vi "itc 503 box controller -- A0.vi"(6 "Log File Path":path, 7 "itc box action":T2=enum."read sweep table", 8 "error in":errorcluster, 9 "Sweep Table In":dbl[][](array[numeric])=[[650.0, 1334.0, 30.0], [300.0, 1334.0, 0.0], [0.0, 0.0, 0.0], [0.0, 0.0, 0.0], [0.0, 0.0, 0.0], [0.0, 0.0, 0.0], [0.0, 0.0, 0.0], [0.0, 0.0, 0.0], [0.0, 0.0, 0.0], [0.0, 0.0, 0.0], [0.0, 0.0, 0.0], [300.0, 0.0, 0.0], [0.0, 0.0, 0.0], [0.0, 0.0, 0.0], [0.0, 0.0, 0.0], [300.0, 0.0, 0.0]], 10 "input":dbl=300.0, 11 "VISA resource name":refnum<visa-resource-name>="GPIB0::23::INSTR") -> (0 "error out":errorcluster, 1 "Sweep Table":dbl[][](array[numeric])=[[650.0, 1334.0, 30.0], [300.0, 1334.0, 0.0], [0.0, 0.0, 0.0], [0.0, 0.0, 0.0], [0.0, 0.0, 0.0], [0.0, 0.0, 0.0], [0.0, 0.0, 0.0], [0.0, 0.0, 0.0], [0.0, 0.0, 0.0], [0.0, 0.0, 0.0], [0.0, 0.0, 0.0], [300.0, 0.0, 0.0], [0.0, 0.0, 0.0], [0.0, 0.0, 0.0], [0.0, 0.0, 0.0], [300.0, 0.0, 0.0]], 2 "itc box state OUT":T1={"ITC503 Address"="GPIB0::15::INSTR", "ITC temperature"=0.0, "ITC set temperature"=300.0, "heater"=300.0, "gas flow"=1.6, "P"=0.0, "D"=10.0, "I"=0.1, "ITC state"="X0A1C2S01H1L0\r", "nonzero temperature"=0.0, "Magn Field (T)"=0.0})   [LabVIEW 2015]
uses:
  itc 503 box - control.ctl
  itc 503 box state.ctl
  Q - not nan -- real.vi
panel:
  out "F-format string":string
  out "enabled state":enum16{"disabled", "enabled"}(ring)
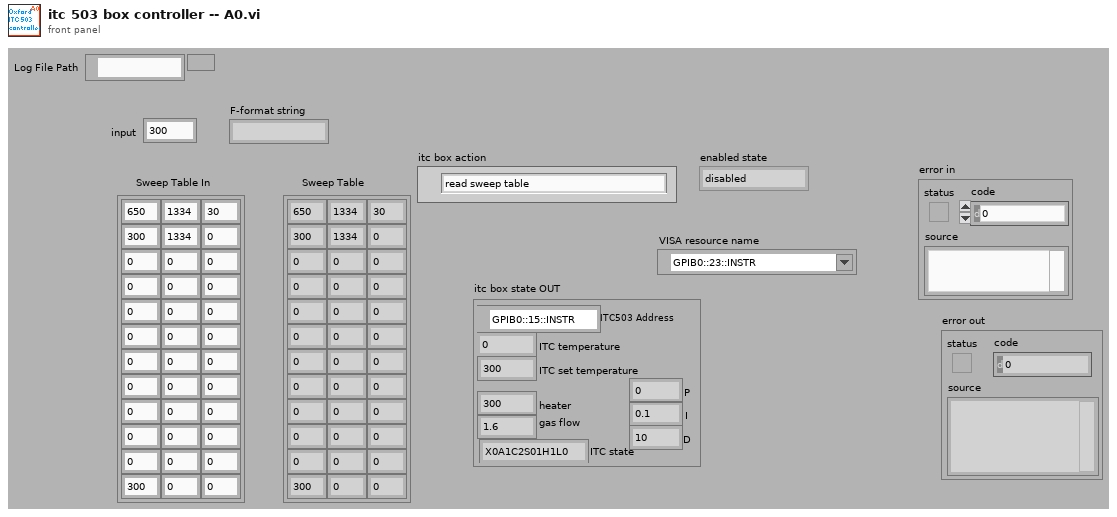
[diagram p1: front panel]
types:
  T1 = typedef "itc 503 box state.ctl" = cluster{"ITC503 Address":refnum<visa-resource-name>, "ITC temperature":dbl, "ITC set temperature":dbl, "heater":dbl, "gas flow":dbl, "P":dbl, "D":dbl, "I":dbl, "ITC state":string, "nonzero temperature":dbl, "Magn Field (T)":dbl}
  T2 = typedef "itc 503 box - control.ctl" = enum16{"heater manual and zero", "heater auto", "upload D", "upload I", "upload P", "shut off", "init", "read sweep table", "disable", "enable", "read state", "set gas to", "stop sweep", "start sweep", "test", "set temperature to", "write sweep table", "-void", "set heater to"}
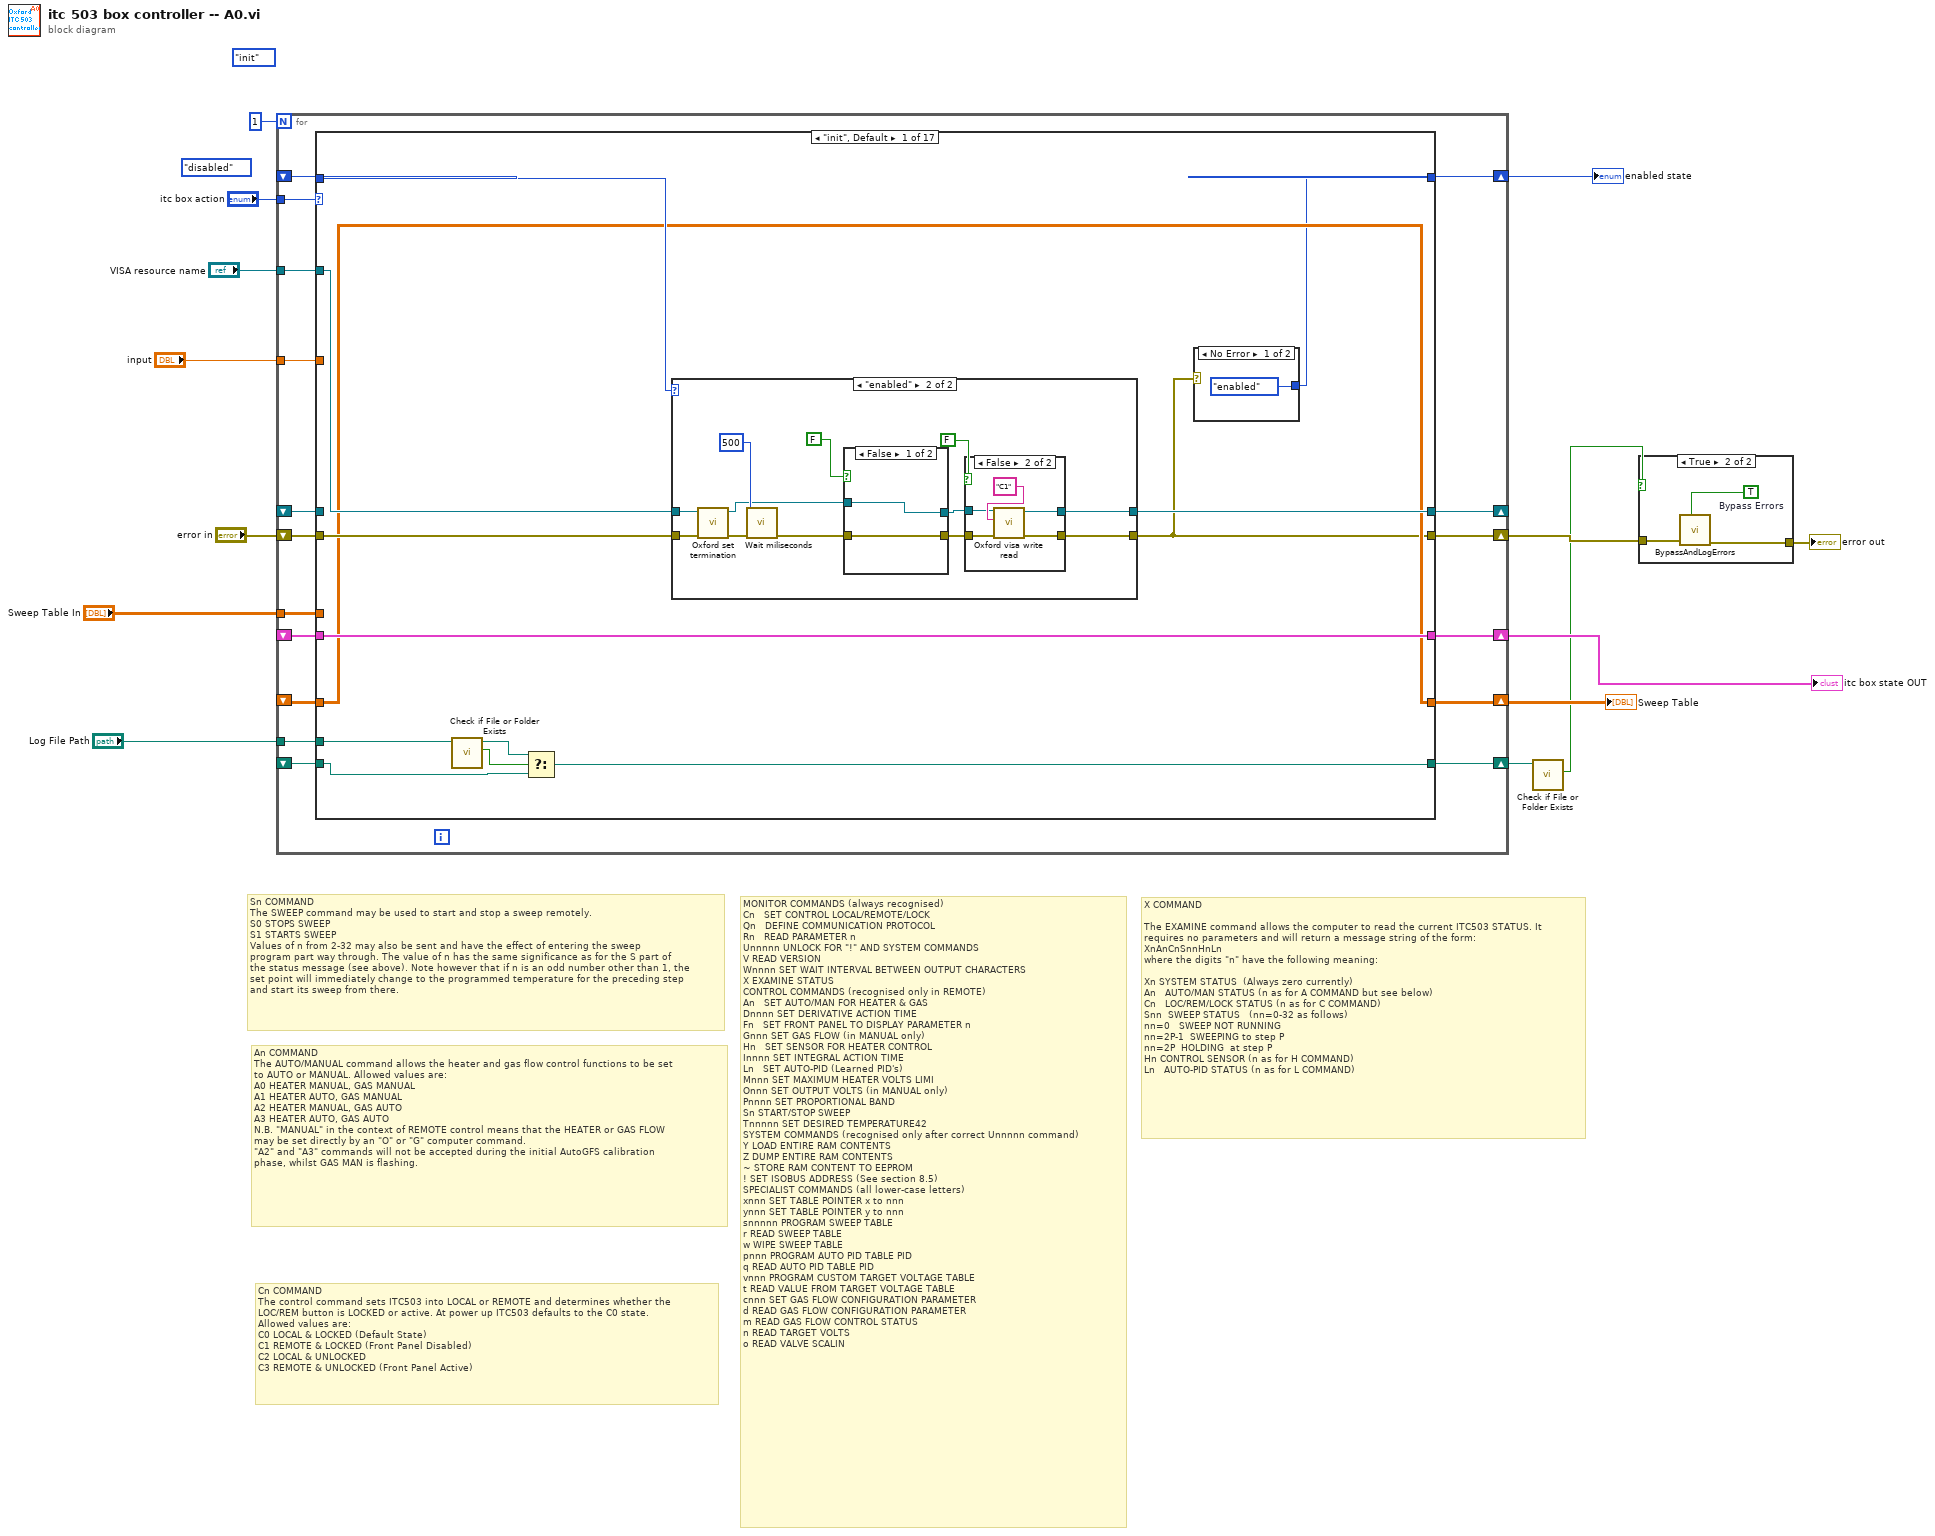
[diagram p0: block diagram]
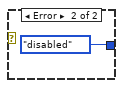
[diagram p3: hidden frame]
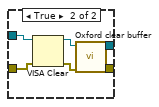
[diagram p5: hidden frame]
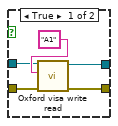
[diagram p6: hidden frame]
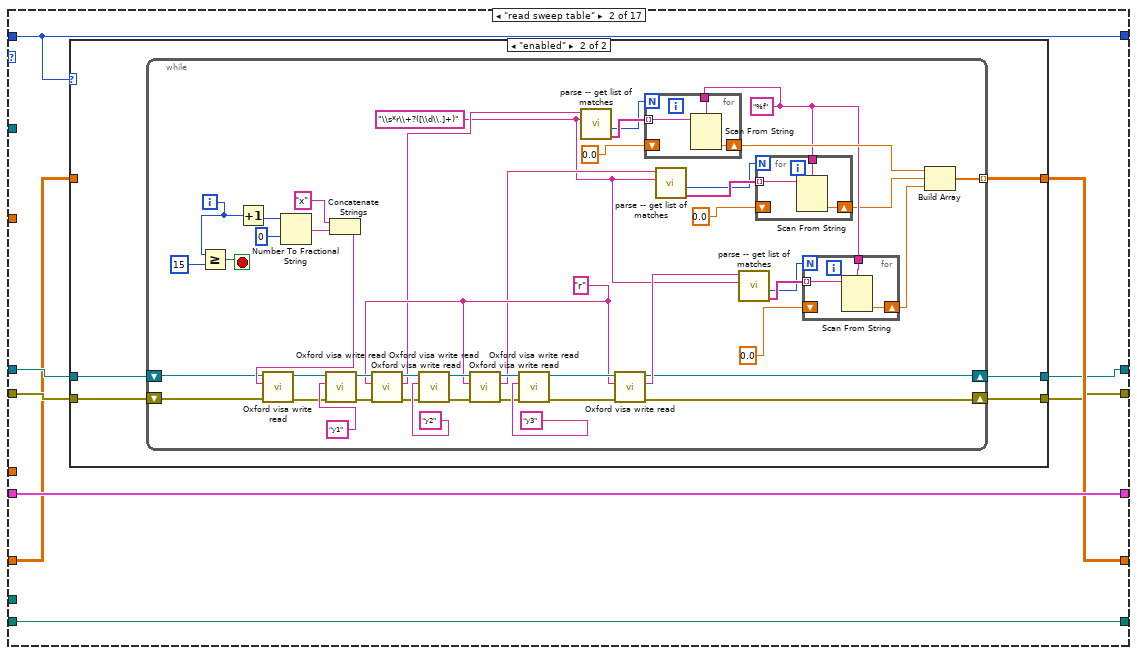
[diagram p7: hidden frame]
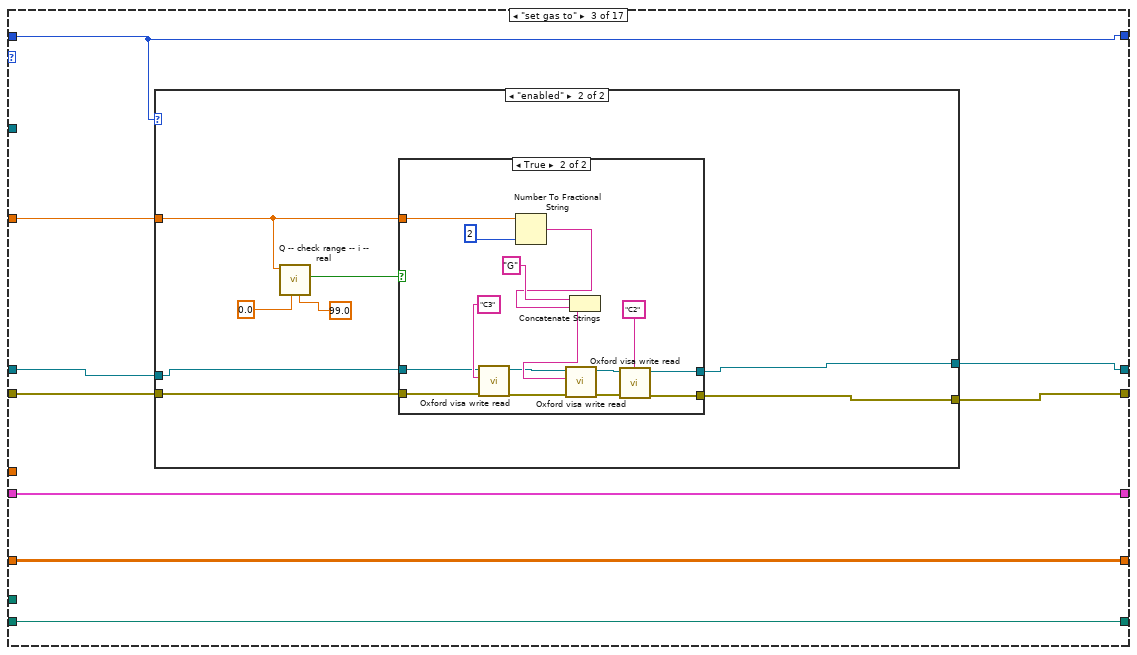
[diagram p9: hidden frame]
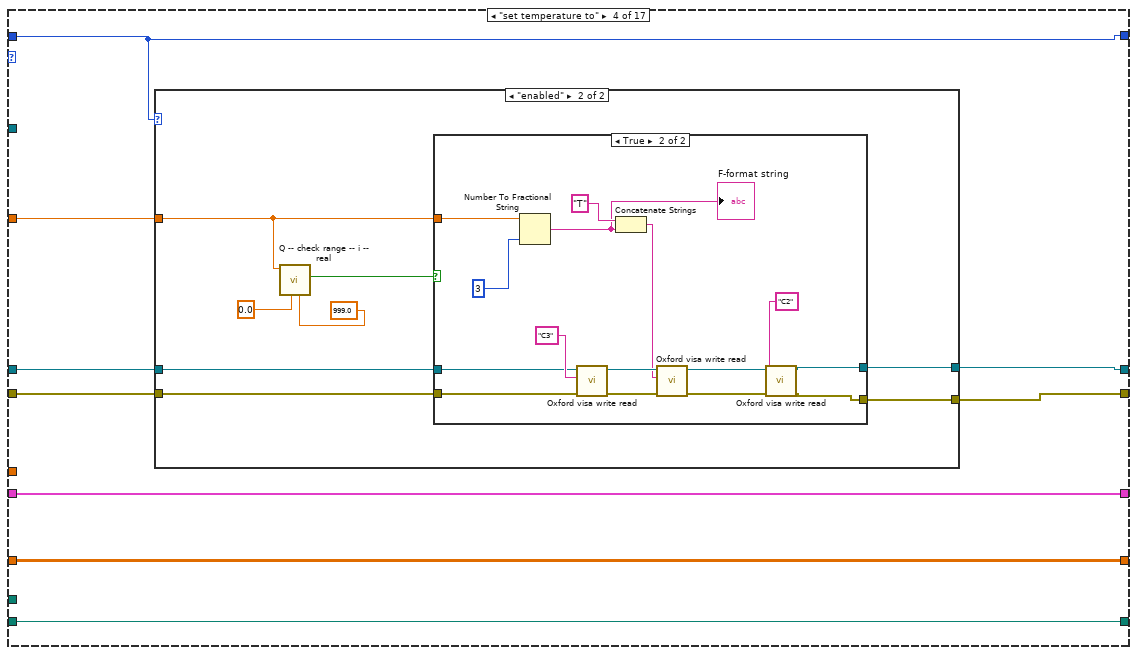
[diagram p12: hidden frame]
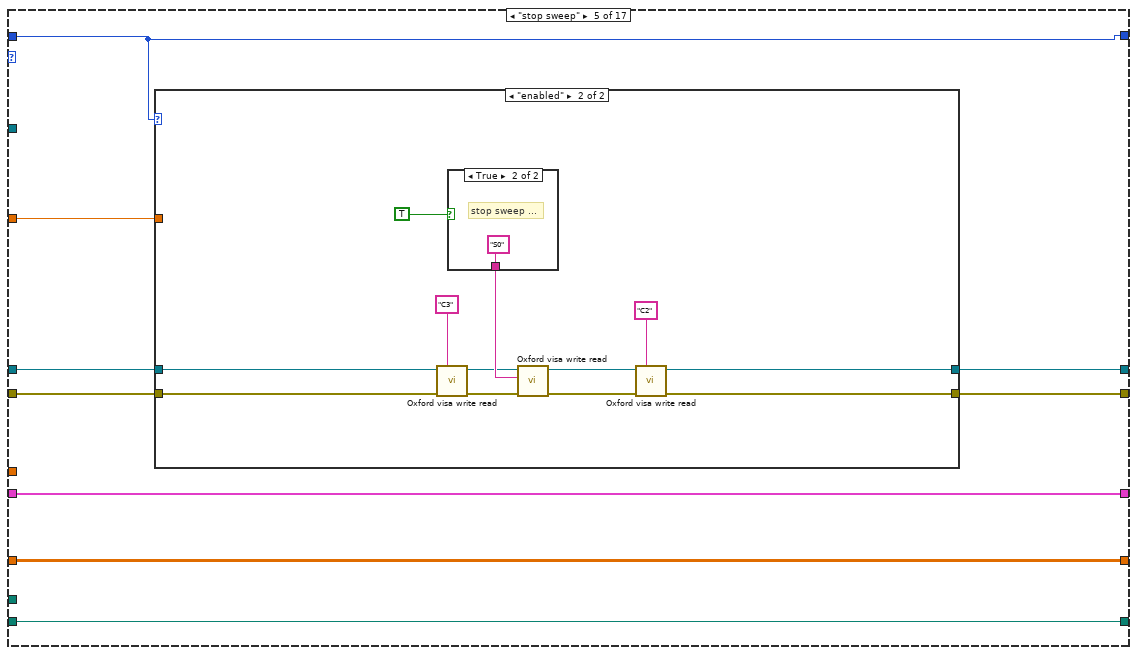
[diagram p15: hidden frame]
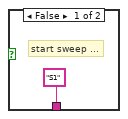
[diagram p17: hidden frame]
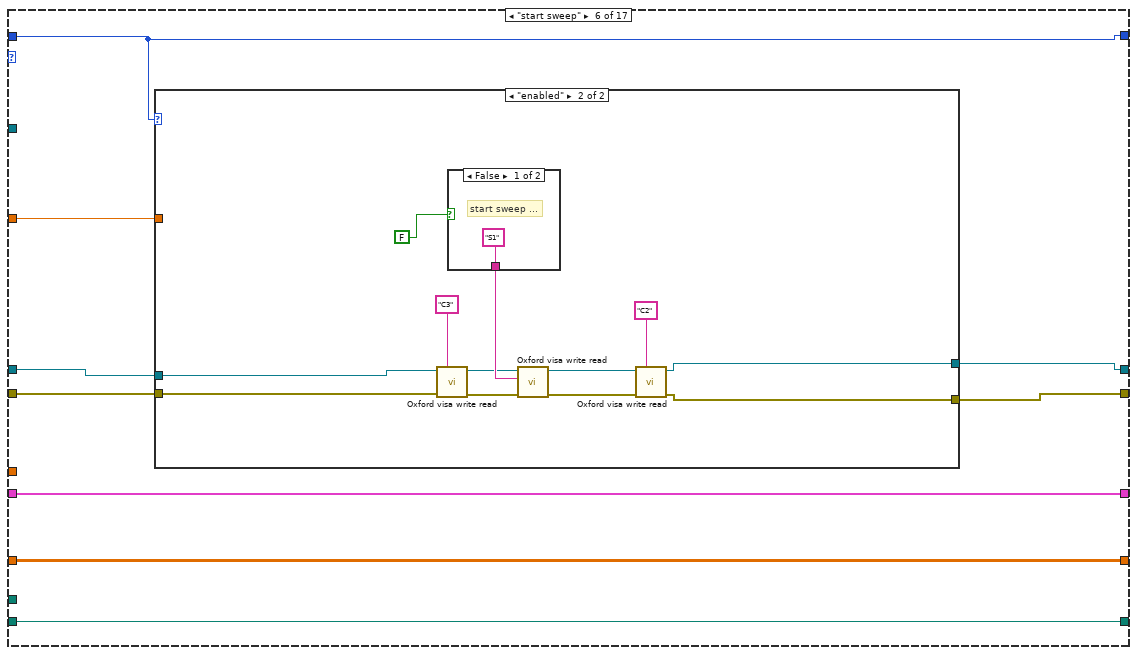
[diagram p18: hidden frame]
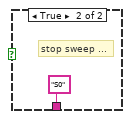
[diagram p20: hidden frame]
diagram:
  (unwired) enum16{"disabled", "enabled"}."disabled" ("disable interaction with itc  2")
  (unwired) itc_503_box_-_control."init" ("itc box action")
  # "Cn COMMAND\nThe control command sets ITC503 into LOCAL or REMOTE and determines whether the\nLOC/REM button is LOCKED or active. At power up ITC503 defaults to the C0 state.\nAllowed values are:\nC0 LOCAL & LOCKED (Default State)\nC1 REMOTE & LOCKED (Front Panel Disabled)\nC2 LOCAL & UNLOCKED\nC3 REMOTE & UNLOCKED (Front Panel Active)"
  # "An COMMAND\nThe AUTO/MANUAL command allows the heater and gas flow control functions to be set\nto AUTO or MANUAL. Allowed values are:\nA0 HEATER MANUAL, GAS MANUAL\nA1 HEATER AUTO, GAS MANUAL\nA2 HEATER MANUAL, GAS AUTO\nA3 HEATER AUTO, GAS AUTO\nN.B. \"MANUAL\" in the context of REMOTE control means that the HEATER or GAS FLOW\nmay be set directly by an \"O\" or \"G\" computer command.\n\"A2\" and \"A3\" commands will not be accepted during the initial AutoGFS calibration\nphase, whilst GAS MAN is flashing."
  # "MONITOR COMMANDS (always recognised)\nCn   SET CONTROL LOCAL/REMOTE/LOCK\nQn   DEFINE COMMUNICATION PROTOCOL\nRn   READ PARAMETER n\nUnnnnn UNLOCK FOR \"!\" AND SYSTEM COMMANDS\nV READ VERSION\nWnnnn SET WAIT INTERVAL BETWEEN OUTPUT CHARACTERS\nX EXAMINE STATUS\nCONTROL COMMANDS (recognised only in REMOTE)\nAn   SET AUTO/MAN FOR HEATER & GAS\nDnnnn SET DERIVATIVE ACTION TIME\nFn   SET FRONT PANEL TO DISPLAY PARAMETER n\nGnnn SET GAS FLOW (in MANUAL only)\nHn   SET SENSOR FOR HEATER CONTROL\nInnnn SET INTEGRAL ACTION TIME\nLn   SET AUTO-PID (Learned PID's)\nMnnn SET MAXIMUM HEATER VOLTS LIMI\nOnnn SET OUTPUT VOLTS (in MANUAL only)\nPnnnn SET PROPORTIONAL BAND\nSn START/STOP SWEEP\nTnnnnn SET DESIRED TEMPERATURE42\nSYSTEM COMMANDS (recognised only after correct Unnnnn command)\nY LOAD ENTIRE RAM CONTENTS\nZ DUMP ENTIRE RAM CONTENTS\n~ STORE RAM CONTENT TO EEPROM\n! SET ISOBUS ADDRESS (See section 8.5)\nSPECIALIST COMMANDS (all lower-case letters)\nxnnn SET TABLE POINTER x to nnn\nynnn SET TABLE POINTER y to nnn\nsnnnnn PROGRAM SWEEP TABLE\nr READ SWEEP TABLE\nw WIPE SWEEP TABLE\npnnn PROGRAM AUTO PID TABLE PID\nq READ AUTO PID TABLE PID\nvnnn PROGRAM CUSTOM TARGET VOLTAGE TABLE\nt READ VALUE FROM TARGET VOLTAGE TABLE\ncnnn SET GAS FLOW CONFIGURATION PARAMETER\nd READ GAS FLOW CONFIGURATION PARAMETER\nm READ GAS FLOW CONTROL STATUS\nn READ TARGET VOLTS\no READ VALVE SCALIN"
  # "X COMMAND\n\nThe EXAMINE command allows the computer to read the current ITC503 STATUS. It\nrequires no parameters and will return a message string of the form:\nXnAnCnSnnHnLn\nwhere the digits \"n\" have the following meaning:\n\nXn SYSTEM STATUS  (Always zero currently)\nAn   AUTO/MAN STATUS (n as for A COMMAND but see below)\nCn   LOC/REM/LOCK STATUS (n as for C COMMAND)\nSnn  SWEEP STATUS   (nn=0-32 as follows)\nnn=0   SWEEP NOT RUNNING\nnn=2P-1  SWEEPING to step P\nnn=2P  HOLDING  at step P\nHn CONTROL SENSOR (n as for H COMMAND)\nLn   AUTO-PID STATUS (n as for L COMMAND)"
  # "Sn COMMAND\nThe SWEEP command may be used to start and stop a sweep remotely.\nS0 STOPS SWEEP\nS1 STARTS SWEEP\nValues of n from 2-32 may also be sent and have the effect of entering the sweep\nprogram part way through. The value of n has the same significance as for the S part of\nthe status message (see above). Note however that if n is an odd number other than 1, the\nset point will immediately change to the programmed temperature for the preceding step\nand start its sweep from there."
  n1 = for {
    N: 1 -> [_]
    tunnel: "itc box action" -> [w31]
    shift-right: [w29] -> _
    shift-left: _ -> [w30]
    tunnel: "VISA resource name" -> [w28]
    shift-right: [w27] -> w7
    shift-left: _ -> [w26]
    shift-right: [w25] -> w6
    shift-left: _ -> [w23]
    shift-right: [w18] -> w4
    shift-left: "error in" -> [w24]
    shift-right: [w22] -> w10
    shift-left: _ -> [w21]
    tunnel: "input" -> [w20]
    tunnel: "Sweep Table In" -> [w19]
    tunnel: "Log File Path" -> [w17]
    shift-right: [w16] -> w2
    shift-left: _ -> [w15]
    n2 = case shown="\"init\", Default" w31 {
      tunnel: w30 -> [_ w85 w158 w194 w230 w255 w280 w306 w332 w358 w380 w405 w449 w461 w478 w542 w548]
      tunnel: [w44 w82 w155 w191 w227 w252 w277 w303 w329 w355 w377 w402 w449 w458 w475 w542 w548] -> w29
      tunnel: w28 -> [w43 _ _ _ _ _ _ _ _ _ _ _ _ _ _ _ _]
      tunnel: [w37 w81 w152 w188 w224 w249 w274 w300 w326 w352 w374 w399 w450 w455 w474 enum16{"disabled", "enabled"}."disabled" ("disable interaction with itc  2") enum16{"disabled", "enabled"}."enabled" ("disable interaction with itc  2")] -> w27
      tunnel: w26 -> [w42 w81 w152 w188 w224 w249 w274 w300 w326 w352 w374 w399 w450 w455 w474 _ _]
      tunnel: [w40 w87 w154 w190 w226 w251 w276 w302 w328 w354 w376 w401 w452 w457 w479 w540 w546] -> w25
      tunnel: w24 -> [w41 w84 w157 w193 w229 w254 w279 w305 w331 w357 w379 w404 w448 w460 w477 w541 w547]
      tunnel: [w38 w83 w156 w192 w228 w253 w278 w304 w330 w356 w378 w403 w448 w459 w476 w541 w547] -> w18
      tunnel: w23 -> [w40 w87 w154 w190 w226 w251 w276 w302 w328 w354 w376 w401 w452 w457 w473 w540 w546]
      tunnel: [w39 w86 w153 w189 w225 w250 w275 w301 w327 w353 w375 w400 w451 w456 w472 w539 w545] -> w22
      tunnel: w21 -> [w39 w80 w153 w189 w225 w250 w275 w301 w327 w353 w375 w400 w451 w456 w472 w539 w545]
      tunnel: w20 -> [_ _ w159 w195 w231 w256 w281 w307 w333 w359 w381 w406 _ w462 _ _ _]
      tunnel: w19 -> [_ _ _ _ _ _ _ _ _ _ _ _ _ w454 _ _ _]
      tunnel: w17 -> [w36 _ _ _ _ _ _ _ _ _ _ _ _ _ _ _ _]
      tunnel: [w33 w79 w151 w187 w223 w248 w273 w299 w325 w351 w373 w398 w447 w453 w471 w538 w544] -> w16
      tunnel: w15 -> [w32 w79 w151 w187 w223 w248 w273 w299 w325 w351 w373 w398 w447 w453 w471 w538 w544]
      frame "init", Default {
        n3 = call <vilib>:"Check if File or Folder Exists.vi"("path"=w36) -> ("file or folder exists?"=w35:bool, "dup path"=w34:path)  [unwired: 8 in, 1 out]
        n4 = Select(t=w34, s=w35, f=w32) -> (s? t:f=w33:path)
        n5 = case shown="\"enabled\"" w42 {
          tunnel: [w48 w57] -> w44
          tunnel: w43 -> [w48 w54]
          tunnel: w41 -> [w47 w53]
          tunnel: [w47 w56] -> w38
          frame "disabled", Default {
          }
          frame "enabled" {
            n6 = call "Oxford set termination.vi"("error in (no error)"=w53, "VISA resource name"=w54) -> ("error out"=w50:errorcluster, "VISA resource name out"=w49:refnum<visa-resource-name>)  [unwired: 8 in]
            n7 = call "Wait miliseconds.vi"("error in (no error)"=w50, "milliseconds to wait"=u32 500) -> ("error out"=w52:errorcluster)  [unwired: 8 in, 1 out]
            n8 = case shown="False" FALSE {
              tunnel: [w61 w68] -> w60
              tunnel: [w62 w67] -> w59
              tunnel: w52 -> [w61 w63]
              tunnel: w49 -> [w62 w66]
              frame False {
              }
              frame True {
                n9 = VISA Clear(VISA resource name=w66, error in (no error)=w63) -> (VISA resource name out=w65:refnum<visa-resource-name>, error out=w64:errorcluster)
                n10 = call "Oxford clear buffer.vi"("error in (no error)"=w64, "VISA resource name"=w65) -> ("error out"=w68:errorcluster, "VISA resource name out"=w67:refnum<visa-resource-name>)  [unwired: 6 in, 2 out]
              }
            }
            n11 = case shown="False" FALSE {
              tunnel: w60 -> [w72 w77]
              tunnel: w59 -> [w71 w76]
              tunnel: [w70 w75] -> w57
              tunnel: [w69 w74] -> w56
              frame True {
                n12 = call "Oxford visa write read.vi"("error in (no error)"=w72, "write buffer"="A1" ("Command"), "VISA resource name"=w71) -> ("error out"=w69:errorcluster, "VISA resource name out"=w70:refnum<visa-resource-name>)  [unwired: 6 in, 1 out]
              }
              frame False {
                n13 = call "Oxford visa write read.vi"("error in (no error)"=w77, "write buffer"="C1" ("Command"), "VISA resource name"=w76) -> ("error out"=w74:errorcluster, "VISA resource name out"=w75:refnum<visa-resource-name>)  [unwired: 6 in, 1 out]
              }
            }
          }
        }
        n14 = case shown="No Error" w38 {
          tunnel: [enum16{"disabled", "enabled"}."enabled" ("disable interaction with itc  2") enum16{"disabled", "enabled"}."disabled" ("disable interaction with itc  2")] -> w37
          frame No Error {
          }
          frame Error {
          }
        }
      }
      frame "read sweep table" {
        n15 = case shown="\"enabled\"" w81 {
          tunnel: [w88 w95] -> w86
          tunnel: w85 -> [w90 w94]
          tunnel: w84 -> [w89 w93]
          tunnel: [w89 w92] -> w83
          tunnel: [w90 w91] -> w82
          tunnel: w80 -> [w88 _]
          frame "disabled", Default {
          }
          frame "enabled" {
            n16 = while {
              tunnel: [w117] -> w95 mode=indexing
              shift-right: [w97] -> w91
              shift-left: w94 -> [w120]
              shift-right: [w96] -> w92
              shift-left: w93 -> [w127]
              i -> [w115]
              stop <- w114 stop-if-true
              w101 = "\\s*r\\+?([\\d\\.]+)" ("format string")
              w100 = "%f" ("format string")
              w119 = "r" ("string")
              n17 = Greater Or Equal?(x=w115, y=15) -> (x >= y?=w114:bool)
              n18 = Increment(x=w115) -> (x+1=w141:i32)
              n19 = Number To Fractional String(number=w141, precision (6)=i16 0) -> (F-format string=w138:string)  [unwired: 2 in]
              n20 = Concatenate Strings("x" ("string"), w138) -> (w137:string)
              n21 = call "Oxford visa write read.vi"("error in (no error)"=w127, "write buffer"=w137, "VISA resource name"=w120) -> ("error out"=w133:errorcluster, "VISA resource name out"=w121:refnum<visa-resource-name>)  [unwired: 6 in, 1 out]
              n22 = call "Oxford visa write read.vi"("error in (no error)"=w133, "write buffer"="y1" ("string"), "VISA resource name"=w121) -> ("error out"=w132:errorcluster, "VISA resource name out"=w122:refnum<visa-resource-name>)  [unwired: 6 in, 1 out]
              n23 = call "Oxford visa write read.vi"("error in (no error)"=w132, "write buffer"=w119, "VISA resource name"=w122) -> ("error out"=w131:errorcluster, "read buffer"=w113:string, "VISA resource name out"=w123:refnum<visa-resource-name>)  [unwired: 6 in]
              n24 = call "Oxford visa write read.vi"("error in (no error)"=w131, "write buffer"="y2" ("string"), "VISA resource name"=w123) -> ("error out"=w130:errorcluster, "VISA resource name out"=w126:refnum<visa-resource-name>)  [unwired: 6 in, 1 out]
              n25 = call "Oxford visa write read.vi"("error in (no error)"=w130, "write buffer"=w119, "VISA resource name"=w126) -> ("error out"=w129:errorcluster, "read buffer"=w102:string, "VISA resource name out"=w125:refnum<visa-resource-name>)  [unwired: 6 in]
              n26 = call "Oxford visa write read.vi"("error in (no error)"=w129, "write buffer"="y3" ("string"), "VISA resource name"=w125) -> ("error out"=w128:errorcluster, "VISA resource name out"=w124:refnum<visa-resource-name>)  [unwired: 6 in, 1 out]
              n27 = call "parse -- get list of matches.vi"("regexp"=w101, "string"=w113) -> ("Array"=w112:string[], "number of free elastic constants"=w111:i32)  [unwired: 7 in, 1 out]
              n28 = call "Oxford visa write read.vi"("error in (no error)"=w128, "write buffer"=w119, "VISA resource name"=w124) -> ("error out"=w96:errorcluster, "read buffer"=w103:string, "VISA resource name out"=w97:refnum<visa-resource-name>)  [unwired: 6 in]
              n29 = for {
                N: w111 -> [_]
                tunnel: w100 -> [w149]
                tunnel: w112 -> [w148] mode=indexing
                shift-right: [w150] -> w118
                shift-left: 0.0 -> [_]
                n30 = Scan From String(format string=w149, input string=w148) -> (output 1=w150:dbl)  [unwired: 3 in, 3 out]
              }
              n31 = call "parse -- get list of matches.vi"("regexp"=w101, "string"=w102) -> ("Array"=w109:string[], "number of free elastic constants"=w108:i32)  [unwired: 7 in, 1 out]
              n32 = call "parse -- get list of matches.vi"("regexp"=w101, "string"=w103) -> ("Array"=w106:string[], "number of free elastic constants"=w105:i32)  [unwired: 7 in, 1 out]
              n33 = for {
                N: w108 -> [_]
                tunnel: w109 -> [w146] mode=indexing
                shift-right: [w147] -> w98
                shift-left: 0.0 -> [_]
                tunnel: w100 -> [w145]
                n34 = Scan From String(format string=w145, input string=w146) -> (output 1=w147:dbl)  [unwired: 3 in, 3 out]
              }
              n35 = for {
                N: w105 -> [_]
                tunnel: w106 -> [w143] mode=indexing
                shift-right: [w144] -> w99
                shift-left: 0.0 -> [_]
                tunnel: w100 -> [w142]
                n36 = Scan From String(format string=w142, input string=w143) -> (output 1=w144:dbl)  [unwired: 3 in, 3 out]
              }
              n37 = Build Array(w118, w98, w99) -> (w117:dbl[])
            }
          }
        }
      }
      frame "set gas to" {
        n38 = case shown="\"enabled\"" w152 {
          tunnel: w159 -> [_ w167]
          tunnel: w158 -> [w161 w165]
          tunnel: w157 -> [w160 w164]
          tunnel: [w160 w163] -> w156
          tunnel: [w161 w162] -> w155
          frame "disabled", Default {
          }
          frame "enabled" {
            n39 = call "Q -- check range -- i -- real.vi"("upper"=99.0, "lower"=0.0, "number"=w167) -> ("in range?"=w166:bool)  [unwired: 6 in, 2 out]
            n40 = case shown="True" w166 {
              tunnel: w164 -> [w171 w178]
              tunnel: [w171 w177] -> w163
              tunnel: [w170 w174] -> w162
              tunnel: w167 -> [_ w173]
              tunnel: w165 -> [w170 w172]
              frame False {
                # "need to rize some kind of error ..."
              }
              frame True {
                n41 = call "Oxford visa write read.vi"("error in (no error)"=w178, "write buffer"="C3" ("Command"), "VISA resource name"=w172) -> ("error out"=w182:errorcluster, "VISA resource name out"=w176:refnum<visa-resource-name>)  [unwired: 6 in, 1 out]
                n42 = Number To Fractional String(number=w173, precision (6)=i16 2) -> (F-format string=w183:string)  [unwired: 2 in]
                n43 = Concatenate Strings("G" ("string"), w183) -> (w180:string)
                n44 = call "Oxford visa write read.vi"("error in (no error)"=w182, "write buffer"=w180, "VISA resource name"=w176) -> ("error out"=w181:errorcluster, "VISA resource name out"=w175:refnum<visa-resource-name>)  [unwired: 6 in, 1 out]
                n45 = call "Oxford visa write read.vi"("error in (no error)"=w181, "write buffer"="C2" ("Command"), "VISA resource name"=w175) -> ("error out"=w177:errorcluster, "VISA resource name out"=w174:refnum<visa-resource-name>)  [unwired: 6 in, 1 out]
              }
            }
          }
        }
      }
      frame "set temperature to" {
        n46 = case shown="\"enabled\"" w188 {
          tunnel: w195 -> [_ w199]
          tunnel: w194 -> [w197 w203]
          tunnel: w193 -> [w196 w198]
          tunnel: [w196 w201] -> w192
          tunnel: [w197 w202] -> w191
          frame "disabled", Default {
          }
          frame "enabled" {
            n47 = call "Q -- check range -- i -- real.vi"("upper"=999.0, "lower"=0.0, "number"=w199) -> ("in range?"=w200:bool)  [unwired: 6 in, 2 out]
            n48 = case shown="True" w200 {
              tunnel: w203 -> [w207 w212]
              tunnel: [w207 w211] -> w202
              tunnel: [w206 w210] -> w201
              tunnel: w199 -> [_ w209]
              tunnel: w198 -> [w206 w208]
              frame False {
              }
              frame True {
                n49 = Number To Fractional String(number=w209, precision (6)=i16 3) -> (F-format string=w217:string)  [unwired: 2 in]
                "F-format string" <- w217
                n50 = call "Oxford visa write read.vi"("error in (no error)"=w208, "write buffer"="C3" ("Command"), "VISA resource name"=w212) -> ("error out"=w222:errorcluster, "VISA resource name out"=w221:refnum<visa-resource-name>)  [unwired: 6 in, 1 out]
                n51 = Concatenate Strings("T" ("Command"), w217) -> (w215:string)
                n52 = call "Oxford visa write read.vi"("error in (no error)"=w222, "write buffer"=w215, "VISA resource name"=w221) -> ("error out"=w213:errorcluster, "VISA resource name out"=w214:refnum<visa-resource-name>)  [unwired: 6 in, 1 out]
                n53 = call "Oxford visa write read.vi"("error in (no error)"=w213, "write buffer"="C2" ("Command"), "VISA resource name"=w214) -> ("error out"=w210:errorcluster, "VISA resource name out"=w211:refnum<visa-resource-name>)  [unwired: 6 in, 1 out]
              }
            }
          }
        }
      }
      frame "stop sweep" {
        n54 = case shown="\"enabled\"" w224 {
          tunnel: w231 -> [_ _]
          tunnel: w230 -> [w233 w234]
          tunnel: w229 -> [w232 w237]
          tunnel: [w232 w236] -> w228
          tunnel: [w233 w235] -> w227
          frame "disabled", Default {
          }
          frame "enabled" {
            n55 = call "Oxford visa write read.vi"("error in (no error)"=w237, "write buffer"="C3" ("Command"), "VISA resource name"=w234) -> ("error out"=w241:errorcluster, "VISA resource name out"=w240:refnum<visa-resource-name>)  [unwired: 6 in, 1 out]
            n56 = case shown="True" TRUE {
              tunnel: ["S1" ("write buffer") "S0" ("write buffer")] -> w245
              frame False {
                # "start sweep ..."
              }
              frame True {
                # "stop sweep ..."
              }
            }
            n57 = call "Oxford visa write read.vi"("error in (no error)"=w241, "write buffer"=w245, "VISA resource name"=w240) -> ("error out"=w244:errorcluster, "VISA resource name out"=w242:refnum<visa-resource-name>)  [unwired: 6 in, 1 out]
            n58 = call "Oxford visa write read.vi"("error in (no error)"=w244, "write buffer"="C2" ("Command"), "VISA resource name"=w242) -> ("error out"=w236:errorcluster, "VISA resource name out"=w235:refnum<visa-resource-name>)  [unwired: 6 in, 1 out]
          }
        }
      }
      frame "start sweep" {
        n59 = case shown="\"enabled\"" w249 {
          tunnel: w256 -> [_ _]
          tunnel: w255 -> [w258 w259]
          tunnel: w254 -> [w257 w262]
          tunnel: [w257 w261] -> w253
          tunnel: [w258 w260] -> w252
          frame "disabled", Default {
          }
          frame "enabled" {
            n60 = call "Oxford visa write read.vi"("error in (no error)"=w262, "write buffer"="C3" ("Command"), "VISA resource name"=w259) -> ("error out"=w266:errorcluster, "VISA resource name out"=w265:refnum<visa-resource-name>)  [unwired: 6 in, 1 out]
            n61 = case shown="False" FALSE {
              tunnel: ["S1" ("write buffer") "S0" ("write buffer")] -> w270
              frame False {
                # "start sweep ..."
              }
              frame True {
                # "stop sweep ..."
              }
            }
            n62 = call "Oxford visa write read.vi"("error in (no error)"=w266, "write buffer"=w270, "VISA resource name"=w265) -> ("error out"=w269:errorcluster, "VISA resource name out"=w267:refnum<visa-resource-name>)  [unwired: 6 in, 1 out]
            n63 = call "Oxford visa write read.vi"("error in (no error)"=w269, "write buffer"="C2" ("Command"), "VISA resource name"=w267) -> ("error out"=w261:errorcluster, "VISA resource name out"=w260:refnum<visa-resource-name>)  [unwired: 6 in, 1 out]
          }
        }
      }
      frame "upload P" {
        n64 = case shown="\"enabled\"" w274 {
          tunnel: w281 -> [_ w284]
          tunnel: w280 -> [w283 w286]
          tunnel: w279 -> [w282 w287]
          tunnel: [w282 w289] -> w278
          tunnel: [w283 w290] -> w277
          frame "disabled", Default {
          }
          frame "enabled" {
            n65 = Number To Fractional String(number=w284, precision (6)=i16 4 ("width (-)")) -> (F-format string=w296:string)  [unwired: 2 in]
            n66 = call "Oxford visa write read.vi"("error in (no error)"=w287, "write buffer"="C3" ("Command"), "VISA resource name"=w286) -> ("error out"=w295:errorcluster, "VISA resource name out"=w292:refnum<visa-resource-name>)  [unwired: 6 in, 1 out]
            n67 = Concatenate Strings("P" ("string"), w296) -> (w298:string)
            n68 = call "Oxford visa write read.vi"("error in (no error)"=w295, "write buffer"=w298, "VISA resource name"=w292) -> ("error out"=w288:errorcluster, "VISA resource name out"=w291:refnum<visa-resource-name>)  [unwired: 6 in, 1 out]
            n69 = call "Oxford visa write read.vi"("error in (no error)"=w288, "write buffer"="C2" ("Command"), "VISA resource name"=w291) -> ("error out"=w289:errorcluster, "VISA resource name out"=w290:refnum<visa-resource-name>)  [unwired: 6 in, 1 out]
          }
        }
      }
      frame "upload I" {
        n70 = case shown="\"enabled\"" w300 {
          tunnel: w307 -> [_ w310]
          tunnel: w306 -> [w309 w312]
          tunnel: w305 -> [w308 w313]
          tunnel: [w308 w315] -> w304
          tunnel: [w309 w316] -> w303
          frame "disabled", Default {
          }
          frame "enabled" {
            n71 = Number To Fractional String(number=w310, precision (6)=i16 4 ("width (-)")) -> (F-format string=w322:string)  [unwired: 2 in]
            n72 = call "Oxford visa write read.vi"("error in (no error)"=w313, "write buffer"="C3" ("Command"), "VISA resource name"=w312) -> ("error out"=w321:errorcluster, "VISA resource name out"=w318:refnum<visa-resource-name>)  [unwired: 6 in, 1 out]
            n73 = Concatenate Strings("I" ("string"), w322) -> (w324:string)
            n74 = call "Oxford visa write read.vi"("error in (no error)"=w321, "write buffer"=w324, "VISA resource name"=w318) -> ("error out"=w314:errorcluster, "VISA resource name out"=w317:refnum<visa-resource-name>)  [unwired: 6 in, 1 out]
            n75 = call "Oxford visa write read.vi"("error in (no error)"=w314, "write buffer"="C2" ("Command"), "VISA resource name"=w317) -> ("error out"=w315:errorcluster, "VISA resource name out"=w316:refnum<visa-resource-name>)  [unwired: 6 in, 1 out]
          }
        }
      }
      frame "upload D" {
        n76 = case shown="\"enabled\"" w326 {
          tunnel: w333 -> [_ w336]
          tunnel: w332 -> [w335 w338]
          tunnel: w331 -> [w334 w339]
          tunnel: [w334 w341] -> w330
          tunnel: [w335 w342] -> w329
          frame "disabled", Default {
          }
          frame "enabled" {
            n77 = Number To Fractional String(number=w336, precision (6)=i16 4 ("width (-)")) -> (F-format string=w348:string)  [unwired: 2 in]
            n78 = call "Oxford visa write read.vi"("error in (no error)"=w339, "write buffer"="C3" ("Command"), "VISA resource name"=w338) -> ("error out"=w347:errorcluster, "VISA resource name out"=w344:refnum<visa-resource-name>)  [unwired: 6 in, 1 out]
            n79 = Concatenate Strings("D" ("string"), w348) -> (w350:string)
            n80 = call "Oxford visa write read.vi"("error in (no error)"=w347, "write buffer"=w350, "VISA resource name"=w344) -> ("error out"=w340:errorcluster, "VISA resource name out"=w343:refnum<visa-resource-name>)  [unwired: 6 in, 1 out]
            n81 = call "Oxford visa write read.vi"("error in (no error)"=w340, "write buffer"="C2" ("Command"), "VISA resource name"=w343) -> ("error out"=w341:errorcluster, "VISA resource name out"=w342:refnum<visa-resource-name>)  [unwired: 6 in, 1 out]
          }
        }
      }
      frame "heater auto" {
        n82 = case shown="\"enabled\"" w352 {
          tunnel: w359 -> [_ _]
          tunnel: w358 -> [w361 w365]
          tunnel: w357 -> [w360 w362]
          tunnel: [w360 w363] -> w356
          tunnel: [w361 w364] -> w355
          frame "disabled", Default {
          }
          frame "enabled" {
            n83 = call "Oxford visa write read.vi"("error in (no error)"=w362, "write buffer"="C3" ("Command"), "VISA resource name"=w365) -> ("error out"=w372:errorcluster, "VISA resource name out"=w370:refnum<visa-resource-name>)  [unwired: 6 in, 1 out]
            n84 = call "Oxford visa write read.vi"("error in (no error)"=w372, "write buffer"="A1" ("Command"), "VISA resource name"=w370) -> ("error out"=w366:errorcluster, "VISA resource name out"=w367:refnum<visa-resource-name>)  [unwired: 6 in, 1 out]
            n85 = call "Oxford visa write read.vi"("error in (no error)"=w366, "write buffer"="C2" ("Command"), "VISA resource name"=w367) -> ("error out"=w363:errorcluster, "VISA resource name out"=w364:refnum<visa-resource-name>)  [unwired: 6 in, 1 out]
          }
        }
      }
      frame "heater manual and zero" {
        n86 = case shown="\"enabled\"" w374 {
          tunnel: w381 -> [_ _]
          tunnel: w380 -> [w383 w387]
          tunnel: w379 -> [w382 w386]
          tunnel: [w382 w385] -> w378
          tunnel: [w383 w384] -> w377
          frame "disabled", Default {
          }
          frame "enabled" {
            n87 = call "Oxford visa write read.vi"("error in (no error)"=w386, "write buffer"="C3" ("Command"), "VISA resource name"=w387) -> ("error out"=w389:errorcluster, "VISA resource name out"=w392:refnum<visa-resource-name>)  [unwired: 6 in, 1 out]
            n88 = call "Oxford visa write read.vi"("error in (no error)"=w389, "write buffer"="A0" ("Command"), "VISA resource name"=w392) -> ("error out"=w388:errorcluster, "VISA resource name out"=w391:refnum<visa-resource-name>)  [unwired: 6 in, 1 out]
            n89 = call "Oxford visa write read.vi"("error in (no error)"=w388, "write buffer"="O000" ("Command"), "VISA resource name"=w391) -> ("error out"=w396:errorcluster, "VISA resource name out"=w395:refnum<visa-resource-name>)  [unwired: 6 in, 1 out]
            n90 = call "Oxford visa write read.vi"("error in (no error)"=w396, "write buffer"="C2" ("Command"), "VISA resource name"=w395) -> ("error out"=w385:errorcluster, "VISA resource name out"=w384:refnum<visa-resource-name>)  [unwired: 6 in, 1 out]
          }
        }
      }
      frame "shut off" {
        n91 = case shown="\"enabled\"" w399 {
          tunnel: w406 -> [_ _]
          tunnel: w405 -> [w408 w418]
          tunnel: w404 -> [w407 w417]
          tunnel: [w407 w416] -> w403
          tunnel: [w408 w415] -> w402
          frame "disabled", Default {
          }
          frame "enabled" {
            w414 = 1.0  # Gas %
            # "stop sweep"
            # "Heater V = 0"
            # "Heater Manual"
            # "Remote"
            n92 = for {
              tunnel: string[] ["C3", "A0", "S0", "O000"] -> [w445] mode=indexing
              shift-right: [w443] -> w413
              shift-left: w418 -> [w446]
              shift-right: [w442] -> w412
              shift-left: w417 -> [w444]
              n93 = call "Oxford visa write read.vi"("error in (no error)"=w444, "write buffer"=w445, "VISA resource name"=w446) -> ("error out"=w442:errorcluster, "VISA resource name out"=w443:refnum<visa-resource-name>)  [unwired: 6 in, 1 out]
            }
            n94 = case shown="True" TRUE {
              tunnel: w412 -> [w421 w428]
              tunnel: [w421 w427] -> w410
              tunnel: [w420 w424] -> w411
              tunnel: w413 -> [w420 w423]
              tunnel: w414 -> [_ w422]
              frame False {
                # "need to rize some kind of error ..."
              }
              frame True {
                n95 = call "Oxford visa write read.vi"("error in (no error)"=w428, "write buffer"="C3" ("Command"), "VISA resource name"=w423) -> ("error out"=w432:errorcluster, "VISA resource name out"=w426:refnum<visa-resource-name>)  [unwired: 6 in, 1 out]
                n96 = Number To Fractional String(number=w422, precision (6)=i16 2) -> (F-format string=w433:string)  [unwired: 2 in]
                n97 = Concatenate Strings("G" ("string"), w433) -> (w430:string)
                n98 = call "Oxford visa write read.vi"("error in (no error)"=w432, "write buffer"=w430, "VISA resource name"=w426) -> ("error out"=w431:errorcluster, "VISA resource name out"=w425:refnum<visa-resource-name>)  [unwired: 6 in, 1 out]
                n99 = call "Oxford visa write read.vi"("error in (no error)"=w431, "write buffer"="C2" ("Command"), "VISA resource name"=w425) -> ("error out"=w427:errorcluster, "VISA resource name out"=w424:refnum<visa-resource-name>)  [unwired: 6 in, 1 out]
              }
            }
            n100 = disable-structure shown="Disabled" {
              disable-tunnel: w411 -> [w440 _]
              disable-tunnel: w410 -> [w439 _]
              disable-tunnel: [w438 _] -> w415
              disable-tunnel: [w437 _] -> w416
              frame Disabled {
                w441 = "C0"  # write buffer
                # "Local locked"
                n101 = call "Oxford visa write read.vi"("error in (no error)"=w439, "write buffer"=w441, "VISA resource name"=w440) -> ("error out"=w437:errorcluster, "VISA resource name out"=w438:refnum<visa-resource-name>)  [unwired: 6 in, 1 out]
              }
              frame Enabled {
              }
            }
          }
        }
      }
      frame "test" {
      }
      frame "write sweep table" {
        n102 = case shown="\"enabled\"" w455 {
          tunnel: w462 -> [_ w465]
          tunnel: w461 -> [w464 w470]
          tunnel: w460 -> [w463 w469]
          tunnel: [w463 w467] -> w459
          tunnel: [w464 w466] -> w458
          tunnel: w454 -> [_ w468]
          frame "disabled", Default {
          }
          frame "enabled" {
            n103 = call "ITC 503 -- upload sweep table.vi"("error in"=w469, "Start set point"=w465, "Sweep Table"=w468, "ITC503 Address"=w470) -> ("error out"=w467:errorcluster, "ITC503 Address OUT"=w466:refnum<visa-resource-name>)  [unwired: 6 in]
          }
        }
      }
      frame "read state" {
        n104 = case shown="\"enabled\"" w474 {
          tunnel: [w480 w488] -> w479
          tunnel: w478 -> [w482 w487]
          tunnel: w477 -> [w481 w486]
          tunnel: [w481 w485] -> w476
          tunnel: [w482 w483] -> w475
          tunnel: w473 -> [w480 _]
          frame "disabled", Default {
          }
          frame "enabled" {
            w504 = FALSE
            n105 = case shown="True" w504 {
              tunnel: [w532 w536] -> w502
              tunnel: [w531 w535] -> w503
              tunnel: w487 -> [w532 w534]
              tunnel: w486 -> [w531 w533]
              frame False {
              }
              frame True {
                n106 = call "Oxford visa write read.vi"("error in (no error)"=w533, "write buffer"="C3" ("Command"), "VISA resource name"=w534) -> ("error out"=w535:errorcluster, "VISA resource name out"=w536:refnum<visa-resource-name>)  [unwired: 6 in, 1 out]
              }
            }
            n107 = call "Oxford visa write read.vi"("error in (no error)"=w503, "write buffer"="X", "VISA resource name"=w502) -> ("error out"=w498:errorcluster, "read buffer"=w489:string, "VISA resource name out"=w499:refnum<visa-resource-name>)  [unwired: 6 in]
            n108 = call "Oxford Read Channel.vi"("error in (no error)"=w498, "Channel #"=1 ("Sensor #"), "VISA resource name"=w499) -> ("error out"=w505:errorcluster, "Data"=w495:dbl, "VISA resource name out"=w511:refnum<visa-resource-name>)  [unwired: 5 in, 1 out]
            n109 = call "Oxford Read Channel.vi"("error in (no error)"=w505, "Channel #"=0 ("Sensor #"), "VISA resource name"=w511) -> ("error out"=w506:errorcluster, "Data"=w494:dbl, "VISA resource name out"=w512:refnum<visa-resource-name>)  [unwired: 5 in, 1 out]
            n110 = call "Oxford Read Channel.vi"("error in (no error)"=w506, "Channel #"=6 ("Sensor #"), "VISA resource name"=w512) -> ("error out"=w507:errorcluster, "Data"=w493:dbl, "VISA resource name out"=w513:refnum<visa-resource-name>)  [unwired: 5 in, 1 out]
            n111 = call "Oxford Read Channel.vi"("error in (no error)"=w507, "Channel #"=7 ("Sensor #"), "VISA resource name"=w513) -> ("error out"=w508:errorcluster, "Data"=w492:dbl, "VISA resource name out"=w514:refnum<visa-resource-name>)  [unwired: 5 in, 1 out]
            n112 = call "Oxford Read Channel.vi"("error in (no error)"=w508, "Channel #"=8 ("Sensor #"), "VISA resource name"=w514) -> ("error out"=w509:errorcluster, "Data"=w491:dbl, "VISA resource name out"=w515:refnum<visa-resource-name>)  [unwired: 5 in, 1 out]
            n113 = call "Oxford Read Channel.vi"("error in (no error)"=w509, "Channel #"=9 ("Sensor #"), "VISA resource name"=w515) -> ("error out"=w510:errorcluster, "Data"=w490:dbl, "VISA resource name out"=w516:refnum<visa-resource-name>)  [unwired: 5 in, 1 out]
            n114 = call "Oxford Read Channel.vi"("error in (no error)"=w510, "Channel #"=10 ("Sensor #"), "VISA resource name"=w516) -> ("error out"=w501:errorcluster, "Data"=w484:dbl, "VISA resource name out"=w500:refnum<visa-resource-name>)  [unwired: 5 in, 1 out]
            n115 = case shown="True" w504 {
              tunnel: w500 -> [w524 w529]
              tunnel: w501 -> [w525 w528]
              tunnel: [w525 w527] -> w485
              tunnel: [w524 w526] -> w483
              frame False {
              }
              frame True {
                n116 = call "Oxford visa write read.vi"("error in (no error)"=w528, "write buffer"="C2" ("Command"), "VISA resource name"=w529) -> ("error out"=w527:errorcluster, "VISA resource name out"=w526:refnum<visa-resource-name>)  [unwired: 6 in, 1 out]
              }
            }
            n117 = Bundle By Name(cluster=T1 {"ITC503 Address"="GPIB0::15::INSTR", "ITC temperature"=0.0, "ITC set temperature"=0.0, "heater"=0.0, "gas flow"=0.0, "P"=0.0, "D"=0.0, "I"=0.0, "ITC state"="", "nonzero temperature"=0.0, "Magn Field (T)"=0.0} ("itc box state OUT"), "ITC503 Address"=w483, "ITC temperature"=w495, "ITC set temperature"=w494, "heater"=w493, "gas flow"=w492, "P"=w491, "D"=w484, "I"=w490, "ITC state"=w489) -> (w488:T1)
          }
        }
      }
      frame "disable" {
      }
      frame "enable" {
      }
    }
  }
  "itc box state OUT" <- w6
  "Sweep Table" <- w10
  "enabled state" <- w7
  n118 = call <vilib>:"Check if File or Folder Exists.vi"("path"=w2) -> ("file or folder exists?"=w1:bool)  [unwired: 8 in, 2 out]
  n119 = case shown="True" w1 {
    tunnel: w4 -> [w550 w552]
    tunnel: [w550 w551] -> w3
    frame False {
    }
    frame True {
      w553 = TRUE  # Bypass Errors
      n120 = call "BypassAndLogErrors.vi"("Bypass Errors"=w553, "error in (no error)"=w552) -> ("error out"=w551:errorcluster)  [unwired: 9 in]
    }
  }
  "error out" <- w3
